vi "Calibrate VNA.vi"(8 "error in (no error)":errorcluster, 9 "Cal kit type":enum16{"E-CAL", "Mechanical"}(ring), 10 "Calibration mode":enum16{"1 Port", "2  Port", "3 Port", "4 Port"}(ring), 11 "VNA-Keysight PNA in":refnum<class "VNA-Keysight PNA.lvclass">) -> (0 "error out":errorcluster, 3 "VNA-Keysight PNA out":refnum<class "VNA-Keysight PNA.lvclass">)   [LabVIEW 2020, in "VNA-Keysight PNA.lvclass"]
uses:
  VNA-Keysight PNA.lvclass
  C:/Sandbox/Git_Sandbox/WiSpry Test Framework source code (LV20)/WiSpry Test Framework/Instruments/Instrument.lvclass
  Instrument.lvclass/Instrument.ctl
  Instrument.lvclass
  <instrlib>/Keysight PNA Series/Keysight PNA Series.lvlib
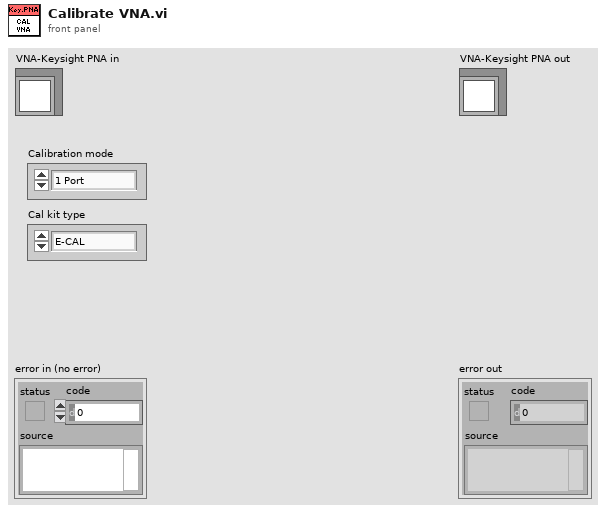
[diagram p1: front panel]
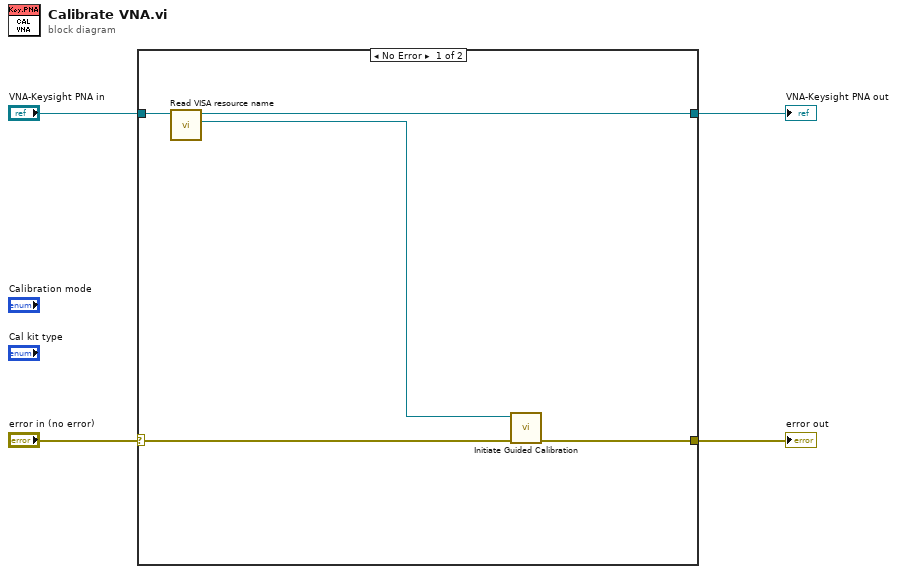
[diagram p0: block diagram]
diagram:
  n1 = case shown="No Error" "error in (no error)" {
    selector: "error in (no error)" -> [w6 w10]
    tunnel: [w8 w11] -> w2
    tunnel: "VNA-Keysight PNA in" -> [w9 w11]
    tunnel: [w7 w10] -> w3
    frame No Error {
      n2 = call "Read VISA resource name.vi"("Instrument in"=w9) -> ("VISA resource name"=w5:refnum<visa-resource-name>, "Instrument out"=w8:refnum<class "VNA-Keysight PNA.lvclass">)  [unwired: 9 in]
      n3 = call <instrlib>:"Initiate Guided Calibration.vi"("error in (no error)"=w6, "VISA resource name"=w5) -> ("error out"=w7:errorcluster)  [unwired: 8 in, 1 out]
    }
    frame Error {
    }
  }
  "error out" <- w3
  "VNA-Keysight PNA out" <- w2
